vi "Measurement.vi"(8 "error in":errorcluster, 11 "User Event References":T2) -> (0 "error out":errorcluster)   [LabVIEW 2015]
uses:
  TypeDef/User Event References.ctl
  TypeDef/GetData Cluster.ctl
  TypeDef/ResultUpdate Cluster.ctl
  TypeDef/Initialize_Cluster.ctl
  TypeDef/OverWrite JSON Cluster.ctl
  <vilib>/event_ctls.llb/usereventprio.ctl
panel:
  out "IsPass":bool=TRUE
  out "Defects":bool[](array[boolean])
  out "Initialize":bool
  out "Measurement is running":bool
  out "tc":u32
  out "Array 1D":dbl[](array[numeric])
  in  "Initialization Values":T1={"InitializationParams"={"CurrentPartNumber"="ECU1512", "MeasurementData"=[{"MeasurementID"=1, "MeasureEnable"=TRUE, "MeasurementPass"=TRUE, "LimitSets"=[{"LimitSetId"=1, "Limits"=[1.5, 2.2]}]}, {"MeasurementID"=2, "MeasureEnable"=TRUE, "MeasurementPass"=TRUE, "LimitSets"=[{"LimitSetId"=1, "Limits"=[1.8, 2.5]}]}, {"MeasurementID"=3, "MeasureEnable"=TRUE, "MeasurementPass"=TRUE, "LimitSets"=[{"LimitSetId"=1, "Limits"=[2.3, 3.2]}]}, {"MeasurementID"=4, "MeasureEnable"=TRUE, "MeasurementPass"=TRUE, "LimitSets"=[{"LimitSetId"=1, "Limits"=[1.6, 2.4]}]}, {"MeasurementID"=5, "MeasureEnable"=TRUE, "MeasurementPass"=TRUE, "LimitSets"=[{"LimitSetId"=1, "Limits"=[2.5, 3.2]}]}]}}
  # "GENERATED DATA Test Bench"
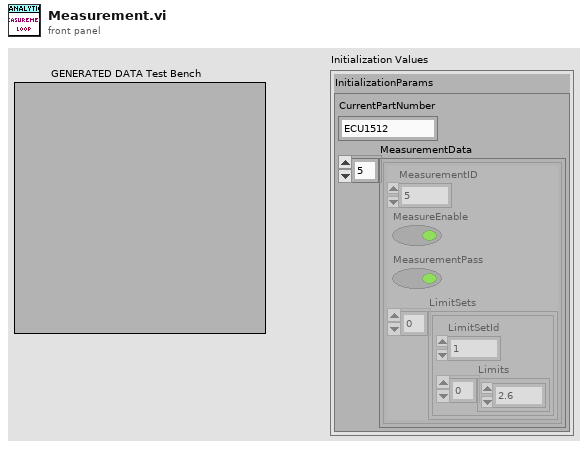
[diagram p1: front panel]
types:
  T1 = cluster{"InitializationParams":cluster{"CurrentPartNumber":string, "MeasurementData":cluster{"MeasurementID":i32, "MeasureEnable":bool, "MeasurementPass":bool, "LimitSets":cluster{"LimitSetId":i32, "Limits":dbl[]}[]}[]}}
  T2 = typedef "User Event References.ctl" = cluster{"Measurement":refnum<user-event>, "Stop_M":refnum<user-event>, "Exit_M":refnum<user-event>, "Analytics":refnum<user-event>, "Back":refnum<user-event>, "Getdata":refnum<user-event>, "ResultUpdate":refnum<user-event>, "Pause_M":refnum<user-event>, "Stop_Analytics":refnum<user-event>, "Exit_Analytics ":refnum<user-event>, "Measurement_M":refnum<user-event>, "Pause_Analytics":refnum<user-event>, "Initialization":refnum<user-event>, "Feedback_Pause":refnum<user-event>, "Feedback_Stop":refnum<user-event>, "Feedback_Exit":refnum<user-event>, "Override JSON":refnum<user-event>}
  T3 = typedef "usereventprio.ctl" = enum32{"high priority", "normal priority"}
  T4 = typedef "ResultUpdate Cluster.ctl" = cluster{"Terminal Count":u32, "isPass":bool, "Terminal Data 1D":dbl[], "Defect":bool[]}
  T5 = typedef "Initialize_Cluster.ctl" = cluster{"Initialization Values ":cluster{"InitializationParams":cluster{"CurrentPartNumber":string, "MeasurementData":cluster{"MeasurementID":i32, "MeasureEnable":bool, "MeasurementPass":bool, "LimitSets":cluster{"LimitSetId":i32, "Limits":dbl[]}[]}[]}}}
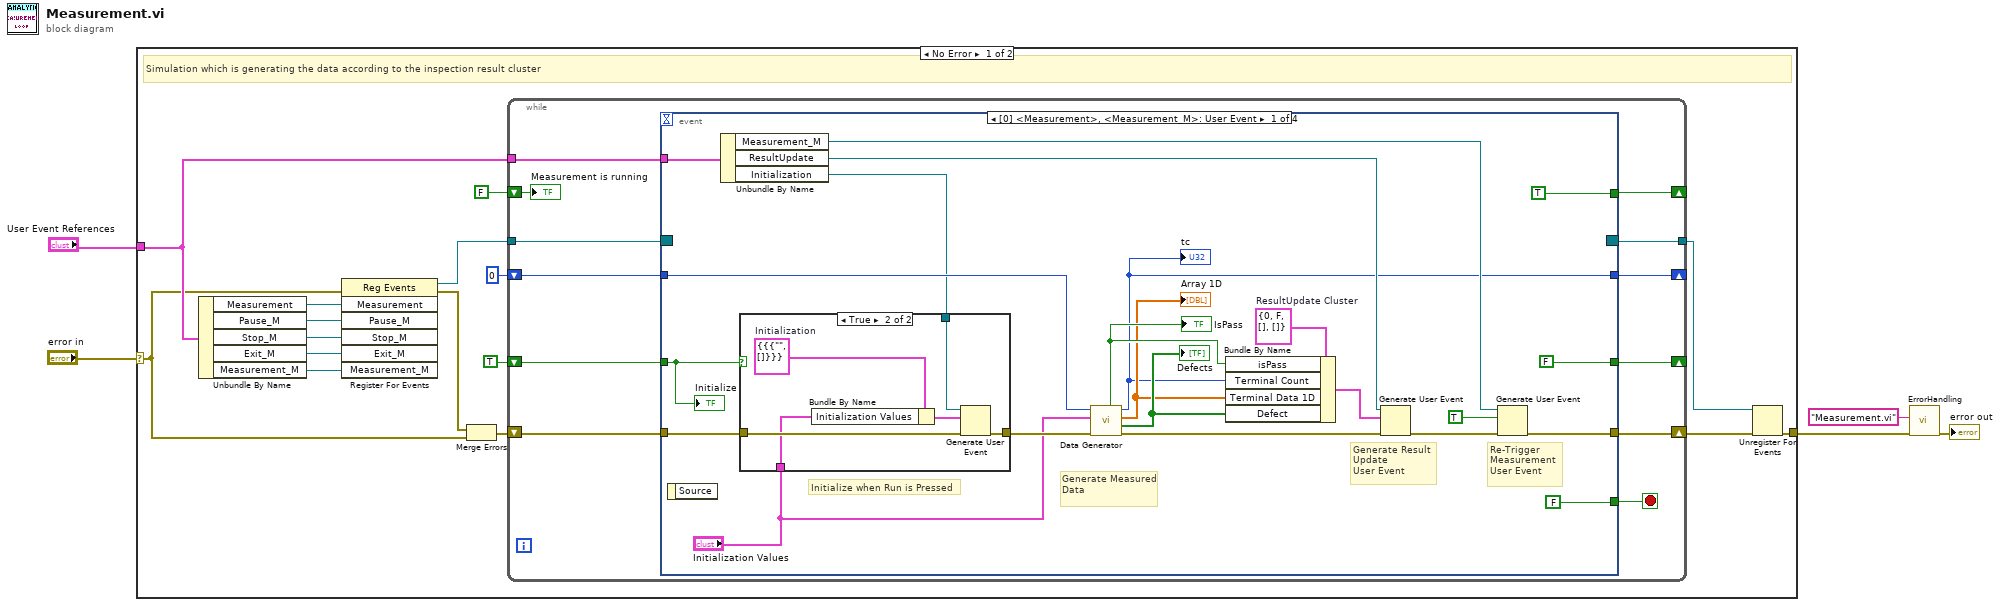
[diagram p0: block diagram]
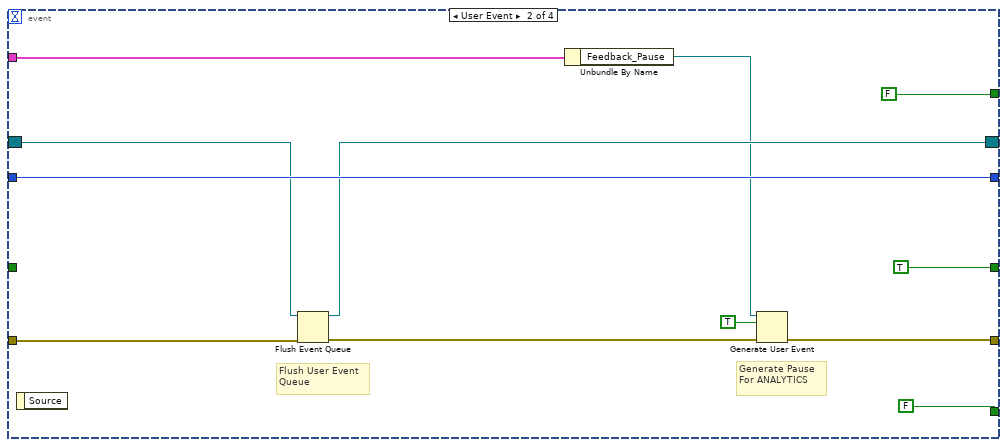
[diagram p3: hidden frame]
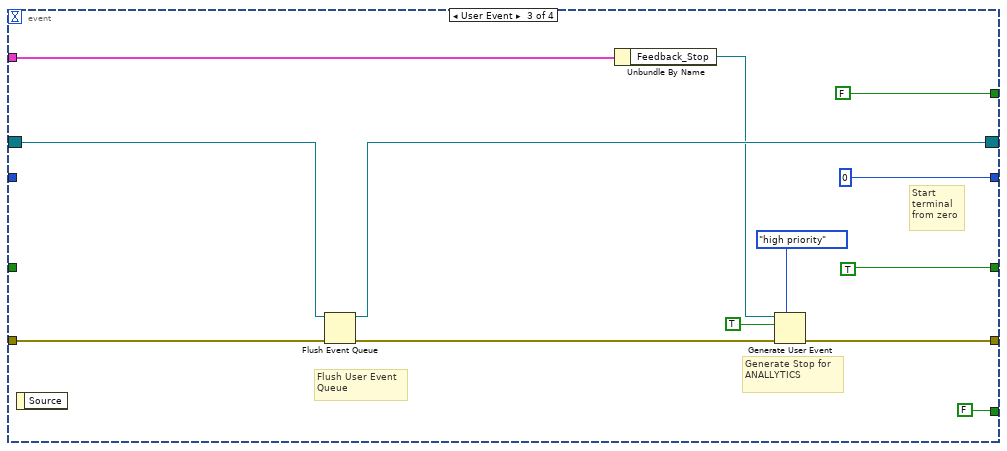
[diagram p4: hidden frame]
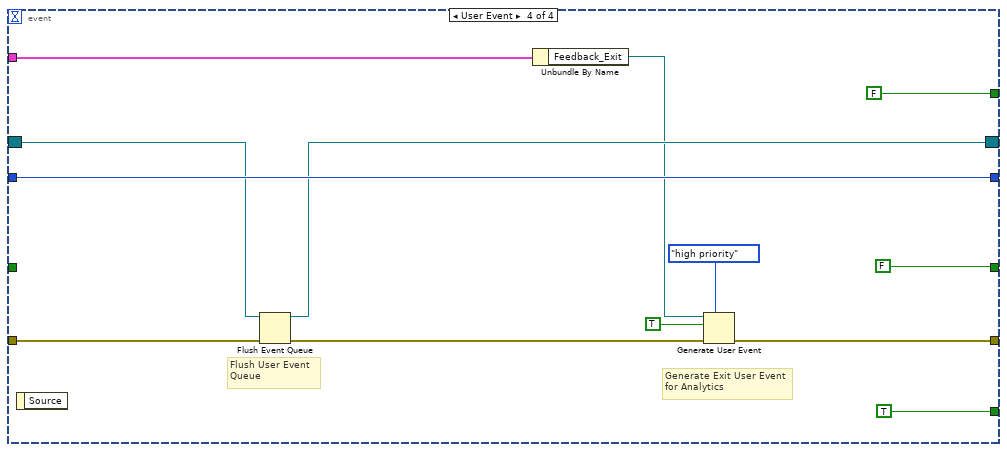
[diagram p5: hidden frame]
diagram:
  n1 = case shown="No Error" "error in" {
    selector: "error in" -> [w6 w101]
    tunnel: "User Event References" -> [w19 _]
    tunnel: [w9 w101] -> w2
    frame No Error {
      # "Simulation which is generating the data according to the inspection result cluster"
      n2 = Unbundle By Name(w19) -> ("Measurement"=w20:refnum<user-event>, "Pause_M"=w16:refnum<user-event>, "Stop_M"=w15:refnum<user-event>, "Exit_M"=w14:refnum<user-event>, "Measurement_M"=w13:refnum<user-event>)
      n3 = register-events(error in=w6, w20, w16, w15, w14, w13) -> (reference out=w21:refnum<event-registration>, error out=w17:errorcluster)  [unwired: 1 in]
      n4 = Merge Errors(w17, w6) -> (w18:errorcluster)
      n5 = while {
        tunnel: w21 -> [w33]
        shift-right: [w29] -> w10
        shift-left: w18 -> [w32]
        shift-right: [w28] -> _
        shift-left: u32 0 ("tc") -> [w31]
        tunnel: w19 -> [w30]
        shift-right: [w26] -> _
        shift-left: FALSE -> [w22]
        tunnel: [w25] -> w8
        shift-right: [w23] -> _
        shift-left: TRUE -> [w24]
        stop <- w27 stop-if-true
        n6 = event shown="[0] <Measurement>, <Measurement_M>: User Event" {
          selector: w33 -> [_ w73 w87 w97]
          dyn-events: [_ w72 w86 w96] -> w25
          timeout: _ -> [_ _ _ _]
          tunnel: w32 -> [w43 w63 w76 w90]
          tunnel: w31 -> [w47 w74 _ w100]
          tunnel: w30 -> [w55 w69 w82 w95]
          tunnel: [w50 w65 w75 w88] -> w29
          tunnel: [w35 w74 u32 0 ("tc") w100] -> w28
          tunnel: [FALSE FALSE FALSE TRUE] -> w27
          tunnel: [TRUE FALSE FALSE FALSE] -> w26
          tunnel: w24 -> [w37 _ _ _]
          tunnel: [FALSE TRUE TRUE FALSE] -> w23
          event User Event {
            w49 = T4 {"Terminal Count"=0, "isPass"=FALSE, "Terminal Data 1D"=[], "Defect"=[]}  # ResultUpdate Cluster
            # "Initialize when Run is Pressed"
            # "Re-Trigger\nMeasurement\nUser Event"
            # "Generate Result Update\nUser Event"
            # "Generate Measured Data"
            n7 = event-data() -> ()  [unwired: 1 in, 1 out]
            n8 = Unbundle By Name(w55) -> ("Measurement_M"=w53:refnum<user-event>, "ResultUpdate"=w54:refnum<user-event>, "Initialization"=w41:refnum<user-event>)
            n9 = case shown="True" w37 {
              tunnel: w43 -> [w56 w62]
              tunnel: [w56 w61] -> w42
              tunnel: w41 -> [_ w60]
              tunnel: "Initialization Values" -> [_ w57]
              frame False {
              }
              frame True {
                w59 = T5 {"Initialization Values "={"InitializationParams"={"CurrentPartNumber"="", "MeasurementData"=[]}}}  # Initialization
                n10 = Bundle By Name(cluster=w59, "Initialization Values"=w57) -> (w58:T5)
                n11 = Generate User Event(user event=w60, event data cluster=w58, error in=w62) -> (error out=w61:errorcluster)  [unwired: 1 in, 1 out]
              }
            }
            n12 = call "Data Generator.vi"("error in"=w42, "Initialization Values"="Initialization Values", "I"=w47) -> ("error out"=w44:errorcluster, "Defects"=w38:bool[], "Values"=w36:dbl[], "tc"=w35:u32, "IsPass"=w39:bool)  [unwired: 4 in]
            "tc" <- w35
            "Array 1D" <- w36
            "Defects" <- w38
            "IsPass" <- w39
            n13 = Bundle By Name(cluster=w49, "isPass"=w39, "Terminal Count"=w35, "Terminal Data 1D"=w36, "Defect"=w38) -> (w48:T4)
            n14 = Generate User Event(user event=w54, event data cluster=w48, error in=w44) -> (error out=w52:errorcluster)  [unwired: 1 in, 1 out]
            n15 = Generate User Event(user event=w53, event data cluster=TRUE, error in=w52) -> (error out=w50:errorcluster)  [unwired: 1 in, 1 out]
            "Initialize" <- w37
          }
          event User Event {
            # "Flush User Event \nQueue"
            # "Generate Pause For ANALYTICS"
            n16 = event-data() -> ()  [unwired: 1 in, 1 out]
            n17 = Flush Event Queue(0:w73, 3:w63) -> (8:w72:refnum<event-registration>, 11:w64:errorcluster)  [unwired: 4 in, 1 out]
            n18 = Unbundle By Name(w69) -> ("Feedback_Pause"=w68:refnum<user-event>)
            n19 = Generate User Event(user event=w68, event data cluster=TRUE, error in=w64) -> (error out=w65:errorcluster)  [unwired: 1 in, 1 out]
          }
          event User Event {
            # "Start terminal from zero"
            # "Flush User Event \nQueue"
            # "Generate Stop for ANALLYTICS"
            n20 = event-data() -> ()  [unwired: 1 in, 1 out]
            n21 = Flush Event Queue(0:w87, 3:w76) -> (8:w86:refnum<event-registration>, 11:w77:errorcluster)  [unwired: 4 in, 1 out]
            n22 = Unbundle By Name(w82) -> ("Feedback_Stop"=w81:refnum<user-event>)
            n23 = Generate User Event(priority (normal)=usereventprio."high priority", user event=w81, event data cluster=TRUE, error in=w77) -> (error out=w75:errorcluster)  [unwired: 1 out]
          }
          event User Event {
            # "Flush User Event \nQueue"
            # "Generate Exit User Event\nfor Analytics"
            n24 = event-data() -> ()  [unwired: 1 in, 1 out]
            n25 = Flush Event Queue(0:w97, 3:w90) -> (8:w96:refnum<event-registration>, 11:w89:errorcluster)  [unwired: 4 in, 1 out]
            n26 = Unbundle By Name(w95) -> ("Feedback_Exit"=w94:refnum<user-event>)
            n27 = Generate User Event(priority (normal)=usereventprio."high priority", user event=w94, event data cluster=TRUE, error in=w89) -> (error out=w88:errorcluster)  [unwired: 1 out]
          }
        }
        "Measurement is running" <- w22
      }
      n28 = Unregister For Events(event registration refnum=w8, error in=w10) -> (error out=w9:errorcluster)
    }
    frame Error {
    }
  }
  n29 = call "ErrorHandling.vi"("error in (no error)"=w2, "Vi-name"="Measurement.vi") -> ("error out"=→"error out":errorcluster)  [unwired: 9 in]
